vi "Calibrate Pseudo-Phasor.vi"(4 "Calibrate(F)/Uncalibrate":bool, 6 "Calibrated Phasor":bool, 8 "Error In":errorcluster, 9 "Target Phasor":cxt, 10 "Calibration Pseudo-Phasor":cxt, 11 "Pseudo-Phasor in":cxt) -> (0 "Error Out":errorcluster, 3 "Pseudo-Phasor out":cxt)   [LabVIEW 2019]
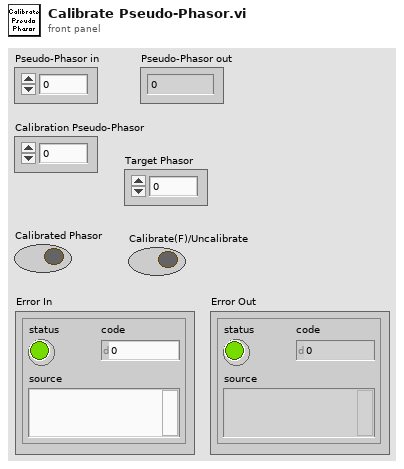
[diagram p1: front panel]
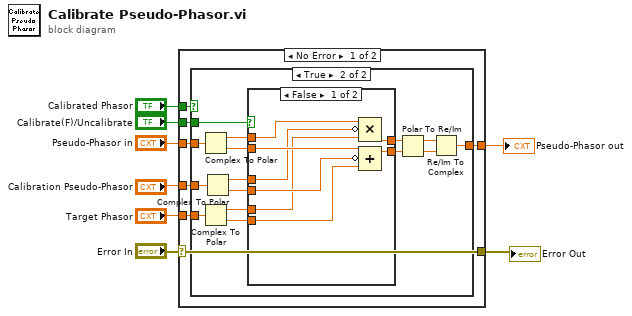
[diagram p0: block diagram]
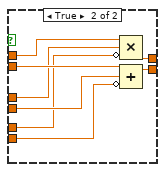
[diagram p3: hidden frame]
diagram:
  n1 = case shown="No Error" "Error In" {
    selector: "Error In" -> [w9 w49]
    tunnel: "Calibration Pseudo-Phasor" -> [w15 _]
    tunnel: "Pseudo-Phasor in" -> [w14 w48]
    tunnel: [w13 w48] -> w6
    tunnel: "Calibrated Phasor" -> [w12 _]
    tunnel: "Target Phasor" -> [w11 _]
    tunnel: "Calibrate(F)/Uncalibrate" -> [w10 _]
    tunnel: [w9 w49] -> w1
    frame No Error {
      n2 = case shown="True" w12 {
        tunnel: w15 -> [_ w31]
        tunnel: w14 -> [w16 w30]
        tunnel: [w16 w27] -> w13
        tunnel: w11 -> [_ w26]
        tunnel: w10 -> [_ w17]
        frame False {
        }
        frame True {
          n3 = Complex To Polar(r * e^(i*theta)=w30) -> (r=w21:ext, theta=w25:ext)
          n4 = Complex To Polar(r * e^(i*theta)=w26) -> (r=w19:ext, theta=w23:ext)
          n5 = Complex To Polar(r * e^(i*theta)=w31) -> (r=w20:ext, theta=w24:ext)
          n6 = case shown="False" w17 {
            tunnel: w25 -> [w39 w47]
            tunnel: w24 -> [w38 w46]
            tunnel: w23 -> [w37 w45]
            tunnel: [w36 w44] -> w22
            tunnel: w21 -> [w35 w43]
            tunnel: w20 -> [w34 w42]
            tunnel: w19 -> [w33 w41]
            tunnel: [w32 w40] -> w18
            frame False {
              n7 = Compound Arithmetic op=MULTIPLY(w35, invert w34, w33) -> (w32:ext)
              n8 = Compound Arithmetic op=ADD(w39, invert w38, w37) -> (w36:ext)
            }
            frame True {
              n9 = Compound Arithmetic op=MULTIPLY(w43, w42, invert w41) -> (w40:ext)
              n10 = Compound Arithmetic op=ADD(w47, w46, invert w45) -> (w44:ext)
            }
          }
          n11 = Polar To Re/Im(2:w22, 3:w18) -> (0:w28:ext, 1:w29:ext)
          n12 = Re/Im To Complex(1:w28, 2:w29) -> (0:w27:cxt)
        }
      }
    }
    frame Error {
    }
  }
  "Pseudo-Phasor out" <- w6
  "Error Out" <- w1
